vi "delete channel none ok.vi"(11 "Indexvals in":u32) -> (2 "Sensor Array out":T1, 3 "Indexvals out":u32)   [LabVIEW 2015]
uses:
  DAQ configuration/Sensor array.ctl
  DAQ configuration/channel identifier.ctl
  DAQ configuration/Sensor buffer command.ctl
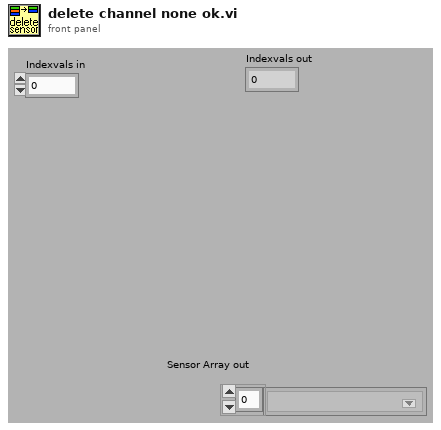
[diagram p1: front panel]
types:
  T1 = typedef "Sensor array.ctl" = T2[]
  T2 = typedef "channel identifier.ctl" = u16
  T3 = typedef "Sensor buffer command.ctl" = enum16{"read average", "read recent", "read all", "write", "set buffer size", "Read channel config", "Write channel config", "clear"}
  T4 = typedef "Channel config.ctl" = cluster{"Channel Indices":T2[], "AI Max voltage":dbl[], "Calibration matrix":T5}
  T5 = typedef "calib array.ctl" = T6[]
  T6 = typedef "conversion.ctl" = cluster{"conversion matrix":sgl[][], "units":string, "name":string, "scale type":T7, "offset (volts)":dbl, "second channel":i8, "correspondence table":T8, "offset (physical units)":dbl, "pH scale":T9, "D.O.":T10, "Photometer data":T11}
  T7 = typedef "scale type.ctl" = enum16{"Volts", "Polynomial", "Correspondence Table", "pH", "Dissolved Oxygen", "Quadratic", "Photometer"}
  T8 = typedef "correspondence table.ctl" = cluster{"physical units":dbl, "volts":dbl}[]
  T9 = typedef "pH scale.ctl" = cluster{"Buffers":cluster{"Buffer":dbl, "Calibrated":bool, "V/T":dbl}[], "Temperature":dbl}
  T10 = typedef "DO scale.ctl" = cluster{"Temperature":dbl, "K":dbl, "barometric pressure":dbl}
  T11 = typedef "Photometer calibration data.ctl" = cluster{"Dark Voltage":dbl, "Blank Voltage":dbl, "Standards":cluster{"Concentration":dbl, "Voltage":dbl}[]}
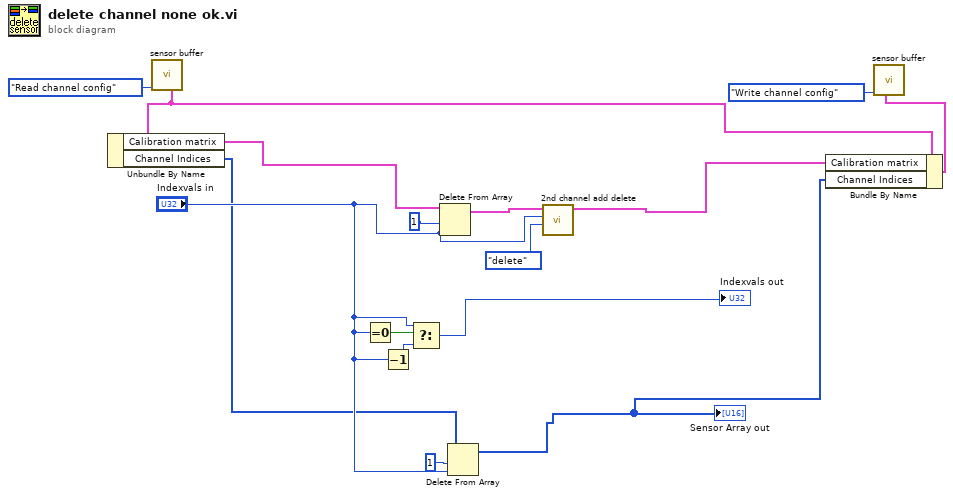
[diagram p0: block diagram]
diagram:
  n1 = call "sensor buffer.vi"("command"=Sensor_buffer_command."Read channel config") -> ("Channel Config out"=w6:T4)  [unwired: 6 in, 4 out]
  n2 = Unbundle By Name(w6) -> ("Calibration matrix"=w2:T5, "Channel Indices"=w1:T2[])
  n3 = Equal To 0?(x="Indexvals in") -> (x = 0?=w10:bool)
  n4 = Decrement(x="Indexvals in") -> (x-1=w9:u32)
  n5 = Select(t="Indexvals in", s=w10, f=w9) -> (s? t:f=→"Indexvals out":u32)
  n6 = Delete From Array(array=w2, length=1 ("Length"), index="Indexvals in") -> (array with subset deleted=w12:T5)  [unwired: 1 out]
  n7 = Delete From Array(array=w1, length=1 ("Length"), index="Indexvals in") -> (array with subset deleted=w3:T2[])  [unwired: 1 out]
  "Sensor Array out" <- w3
  n8 = call "2nd channel add delete.vi"("action"=enum16{"delete", "insert"}."delete", "Index"="Indexvals in", "Calibration array"=w12) -> ("Calibration array out"=w4:T5)  [unwired: 8 in]
  n9 = Bundle By Name(cluster=w6, "Calibration matrix"=w4, "Channel Indices"=w3) -> (w5:T4)
  n10 = call "sensor buffer.vi"("Channel Config"=w5, "command"=Sensor_buffer_command."Write channel config") -> ()  [unwired: 5 in, 5 out]
